vi "Open 2450.vi"() -> (0 "错误输出":errorcluster, 2 "仪器存在":bool, 3 "VISA资源名称输出":refnum<visa-resource-name>)   [LabVIEW 2020]
uses:
  Global variable.vi
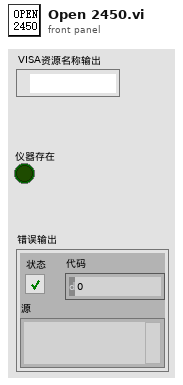
[diagram p1: front panel]
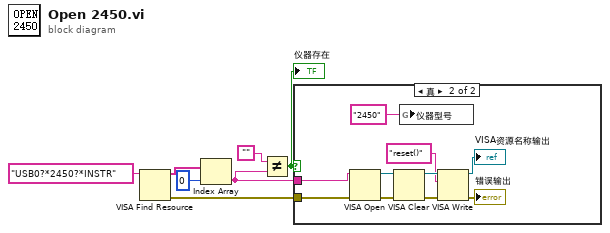
[diagram p0: block diagram]
diagram:
  n1 = VISA Find Resource(11:"USB0?*2450?*INSTR" ("表达式(\"?*\")")) -> (0:w7:errorcluster, 3:w5:string[])  [unwired: 2 in, 1 out]
  n2 = Index Array(array=w5, index=0 ("索引")) -> (element=w3:string)
  n3 = Not Equal?(x="", y=w3) -> (x != y?=w1:bool)
  "仪器存在" <- w1
  n4 = case shown="真" w1 {
    tunnel: w7 -> [_ w10]
    tunnel: w3 -> [_ w9]
    frame False {
    }
    frame True {
      n5 = VISA Open(error in (no error)=w10, VISA resource name=w9) -> (VISA resource name=w17:refnum<visa-resource-name>, error out=w16:errorcluster)  [unwired: 3 in]
      n6 = VISA Clear(VISA resource name=w17, error in (no error)=w16) -> (VISA resource name out=w15:refnum<visa-resource-name>, error out=w14:errorcluster)
      n7 = global write "Global variable.vi" "仪器型号"("2450") -> ()
      n8 = VISA Write(VISA resource name=w15, write buffer="reset()" ("写入缓冲区"), error in (no error)=w14) -> (VISA resource name out=→"VISA资源名称输出":refnum<visa-resource-name>, error out=→"错误输出":errorcluster)  [unwired: 1 out]
    }
  }
